vi "Force Flight Mode.vi"(7 "Timeout (s)":dbl=10.0, 8 "Error In":errorcluster, 11 "Aircraft Mode":T1=enum."LOITER") -> (0 "Error Out":errorcluster, 3 "reset button state":bool)   [LabVIEW 2014]
uses:
  MAVLink/Controls/MAVLink Flight modes.ctl
  <vilib>/Platform/TimedLoop/XDataNode/timing_clust.ctl
  <vilib>/Platform/TimedLoop/XDataNode/nitl_modes.ctl
  <vilib>/Platform/TimedLoop/XDataNode/wakeup.ctl
  Aircraft Information/Sub VI/Get Aircraft Information.vi
  <vilib>/platform/TimedLoop/XDataNode/XDataNode.xnode
  <vilib>/Platform/TimedLoop/XDataNode/XDNodeRunTimeDep.lvlib
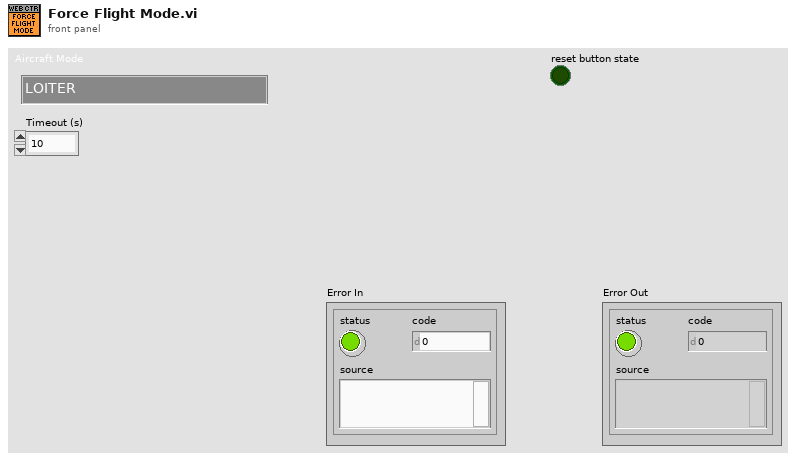
[diagram p1: front panel]
types:
  T1 = typedef "MAVLink Flight modes.ctl" = enum32{"STABILISE", "ACRO", "ALT HOLD", "AUTO", "GUIDED", "LOITER", "RTL", "CIRCLE", "UNKNOWN1", "LAND", "OF LOITER", "DRIFT", "UNKNOWN2", "SPORT", "FLIP", "AUTO TUNE", "POS HOLD", "BRAKE"}
  T2 = typedef "XDNodeRunTimeDep.lvlib/timing_clust.ctl" = cluster{"Expected End [f-1]":u64, "Actual End [f-1]":u64, "Finished Late? [f-1]":bool, "Expected End [i-1]":u64, "Actual End [i-1]":u64, "Finished Late? [i-1]":bool, "Expected Start [i]":u64, "Actual Start [i]":u64, "Expected Start [f]":u64, "Actual Start [f]":u64, "Source Name":string, "Structure Name":string, "Period":i64, "Deadline":i64, "Offset":i64, "Start":i64, "Priority":i32, "Timeout":i32, "Mode":T3, "Wakeup Reason":T4, "Error":errorcluster, "Source Type":string, "Secondary Source Type":string, "Global End Time":u64, "Global Start Time":u64, "Frame Duration":u64, "Iteration Duration":u64, "Assigned CPU":i32, "I/O Scan Engine Mode":u32}
  T3 = typedef "XDNodeRunTimeDep.lvlib/nitl_modes.ctl" = enum32{"No Change", "Process missed periods, maintain original phase", "Discard missed periods, maintain original phase", "Process missed periods, ignore original phase", "Discard missed periods, ignore original phase"}
  T4 = typedef "XDNodeRunTimeDep.lvlib/wakeup.ctl" = enum32{"Normal", "Aborted", "Asynchronous wakeup", "Timing source error", "Timed loop error", "Timeout"}
  T5 = typedef "Drone Information.ctl" = cluster{"Aircraft ID":u8, "Tag ID":string, "System Status":string, "Base Mode":T6, "Armed/Disarmed":bool, "Battery Voltage":dbl, "Control Mode":T7, "Initialisation":u8, "Coms with aircraft good":bool, "Mode":string, "Mission Uploaded":bool}
  T6 = typedef "Base Mode.ctl" = cluster{"Custom Mode":bool, "Test Enabled":bool, "Autonomous Mode":bool, "Guided Mode":bool, "Stabilization Enabled":bool, "HIL Enabled":bool, "Manual Mode":bool, "Arm":bool}
  T7 = typedef "Aircraft Mode.ctl" = enum16{"Loiter", "Stabalise", "Failsafe", "Emergency Stop"}
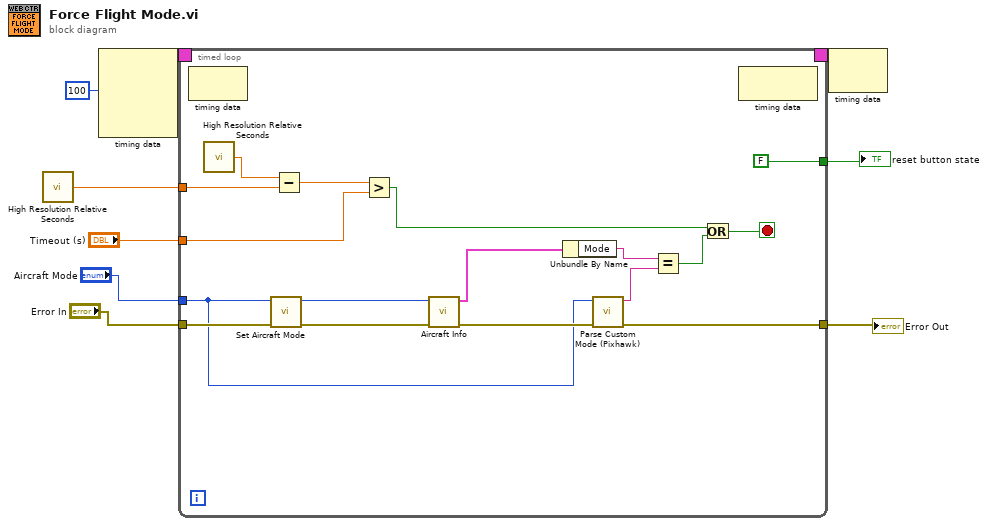
[diagram p0: block diagram]
diagram:
  n1 = call <vilib>:"High Resolution Relative Seconds.vi"() -> ("relative seconds"=w7:dbl)
  n2 = node-c288(i64 100 ("Period")) -> (w9:T2)  [unwired: 3 in]
  n3 = timed-loop {
    timing: w9 -> [_]
    timing-out: [_] -> w8
    tunnel: w7 -> [w25]
    tunnel: "Error In" -> [w24]
    tunnel: "Aircraft Mode" -> [w20]
    tunnel: [w16] -> w3
    tunnel: "Timeout (s)" -> [w13]
    tunnel: [FALSE] -> w1
    stop <- w11 stop-if-true
    n4 = node-c288() -> ()  [unwired: 1 in, 1 out]
    n5 = call <vilib>:"High Resolution Relative Seconds.vi"() -> ("relative seconds"=w26:dbl)
    n6 = call "Set Aircraft Mode.vi"("Error In"=w24, "Aircraft Mode"=w20) -> ("error out"=w22:errorcluster, "Selected Aircraft ID Out"=w23:u8)  [unwired: 8 in]
    n7 = Subtract(x=w26, y=w25) -> (x-y=w14:dbl)
    n8 = Greater?(x=w14, y=w13) -> (0:w12:bool)
    n9 = call-poly "Aircraft Info.vi"("Error In"=w22, "Aircraft ID"=w23) -> ("Error Out"=w21:errorcluster, "Aircraft Information Out"=w19:T5)  [unwired: 8 in]
    n10 = Unbundle By Name(w19) -> ("Mode"=w18:string)
    n11 = call "Parse Custom Mode (Pixhawk).vi"("Error In"=w21, "custom mode"=w20) -> ("Error Out"=w16:errorcluster, "Custom Mode"=w17:string)  [unwired: 8 in]
    n12 = Equal?(x=w18, y=w17) -> (x = y?=w15:bool)
    n13 = Or(x=w12, y=w15) -> (x .or. y?=w11:bool)
    n14 = node-c288() -> ()  [unwired: 1 in, 1 out]
  }
  "Error Out" <- w3
  "reset button state" <- w1
  n15 = node-c288(w8) -> ()  [unwired: 1 out]
